vi "Get Waveform.vi"(8 "error in (no error)":errorcluster, 9 "Post-trigger points":i32, 10 "Pre-trigger points":i32, 11 "RP Instrument in":refnum<class "RP Instrument.lvclass">) -> (0 "error out":errorcluster, 2 "Data out":i16[](array[numeric]), 3 "RP Instrument out":refnum<class "RP Instrument.lvclass">)   [LabVIEW 2015, in "RP Instrument.lvclass"]
uses:
  RP Instrument.lvclass
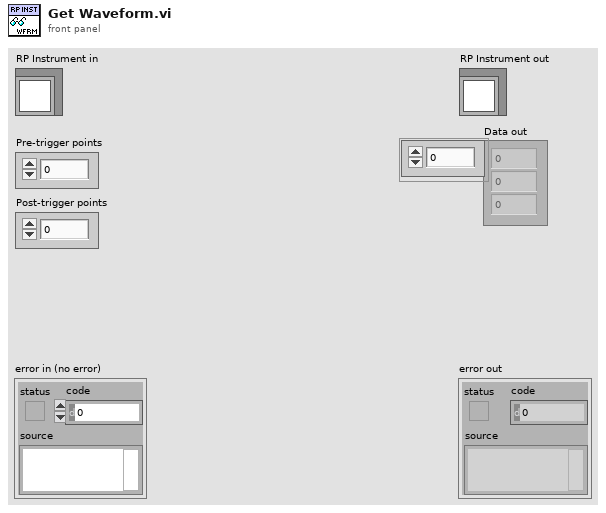
[diagram p1: front panel]
types:
  T1 = enum16{"big-endian, network order", "native, host order", "little-endian"}
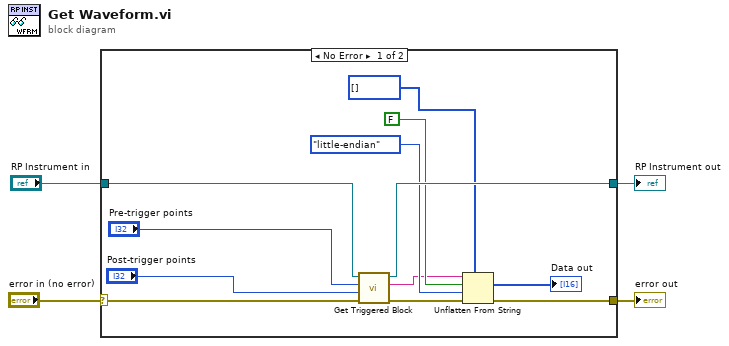
[diagram p0: block diagram]
diagram:
  n1 = case shown="No Error" "error in (no error)" {
    selector: "error in (no error)" -> [w16 w18]
    tunnel: [w10 w18] -> w3
    tunnel: [w15 w17] -> w1
    tunnel: "RP Instrument in" -> [w6 w17]
    frame No Error {
      n2 = call-dynamic "Get Triggered Block.vi"("error in (no error)"=w16, "Post-trigger points"="Post-trigger points", "Pre-trigger points"="Pre-trigger points", "RP Instrument in"=w6) -> ("error out"=w11:errorcluster, "Data out"=w9:string, "RP Instrument out"=w15:refnum<class "RP Instrument.lvclass">)  [unwired: 5 in]
      n3 = Unflatten From String(type=i16[] [], binary string=w9, data includes array or string size? (T)=FALSE, byte order (0:big-endian, network order)=T1."little-endian", error in (no error)=w11) -> (value=→"Data out":i16[], error out=w10:errorcluster)  [unwired: 1 out]
    }
    frame Error {
    }
  }
  "error out" <- w3
  "RP Instrument out" <- w1
